vi "CameraSetupKineticSeries.vi"(1 "kinetic series pars":T1, 2 "subimage cluster":T2, 3 "error in (no error)":errorcluster, 4 "EM adv":bool) -> (5 "actual EM gain":i32, 6 "image size":cluster{"xpixels":i32, "ypixels":i32}, 7 "error out":errorcluster)   [LabVIEW 2019]
uses:
  <userlib>/atmcd32d.llb/TriggerMode_mode typedef.ctl
  <userlib>/atmcd32d.llb/AcquisitionMode_mode typedef.ctl
  <userlib>/atmcd32d.llb/ReadMode_mode typedef.ctl
  <userlib>/atmcd32d.llb/HSSpeed_type typedef.ctl
  <userlib>/atmcd32d.llb/EMGainMode_mode typedef.ctl
  GlobalCamSettingsExperiment.vi
  Global.lvlib
panel:
  out "DLL error code":u32
  out "kinetic":sgl format="%.5f"
  out "accumulate":sgl format="%.2f"
  out "exposure":sgl format="%.5f"
  out "EM gain max":i32
  out "EM gain min":i32
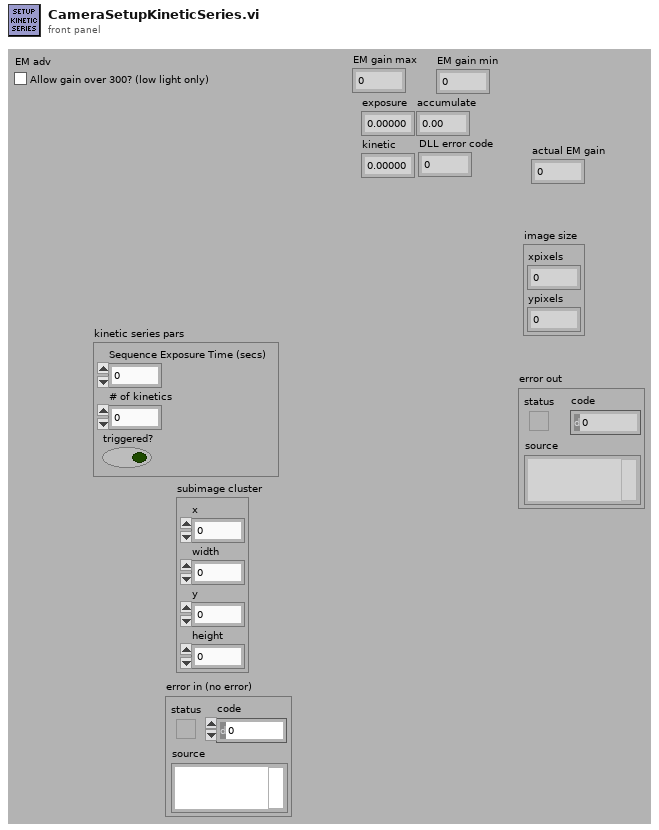
[diagram p1: front panel]
types:
  T1 = cluster{"Sequence Exposure Time (secs)":sgl, "# of kinetics":i32, "triggered?":bool}
  T2 = cluster{"x":i32, "width":i32, "y":i32, "height":i32}
  T3 = typedef "TriggerMode_mode typedef.ctl" = enum16{"Internal", "External", "N/A (2)", "N/A (3)", "N/A (4)", "N/A (5)", "External Start", "External Exposure (Bulb)", "N/A (8)", "External FVB EM", "Software", "N/A (11)", "External Charge Shifting"}
  T4 = typedef "ReadMode_mode typedef.ctl" = enum16{"Full Vertical Binning", "Multi-Track", "Random-Track", "Single-Track", "Image"}
  T5 = typedef "AcquisitionMode_mode typedef.ctl" = enum16{"Reserved (0)", "Single Scan", "Accumulate", "Kinetics", "Fast Kinetics", "Run Till Abort", "Reserved (6)", "Reserved (7)", "Reserved (8)", "Time Delayed Integration"}
  T6 = typedef "CameraSettings.ctl" = cluster{"EM Gain :":dbl, "Pre Amp Gain :":dbl, "VS Speed [Index] :":dbl, "VS Amplitude :":dbl, "Exposure Time [s] :":dbl, "Temperature :":dbl, "HS Speed [s]":dbl, "Gain > 300 :":bool}
  T7 = typedef "HSSpeed_type typedef.ctl" = enum16{"EM Amp", "Conventional Amp"}
  T8 = typedef "EMGainMode_mode typedef.ctl" = enum16{"8-bit", "12-bit", "Linear", "Real"}
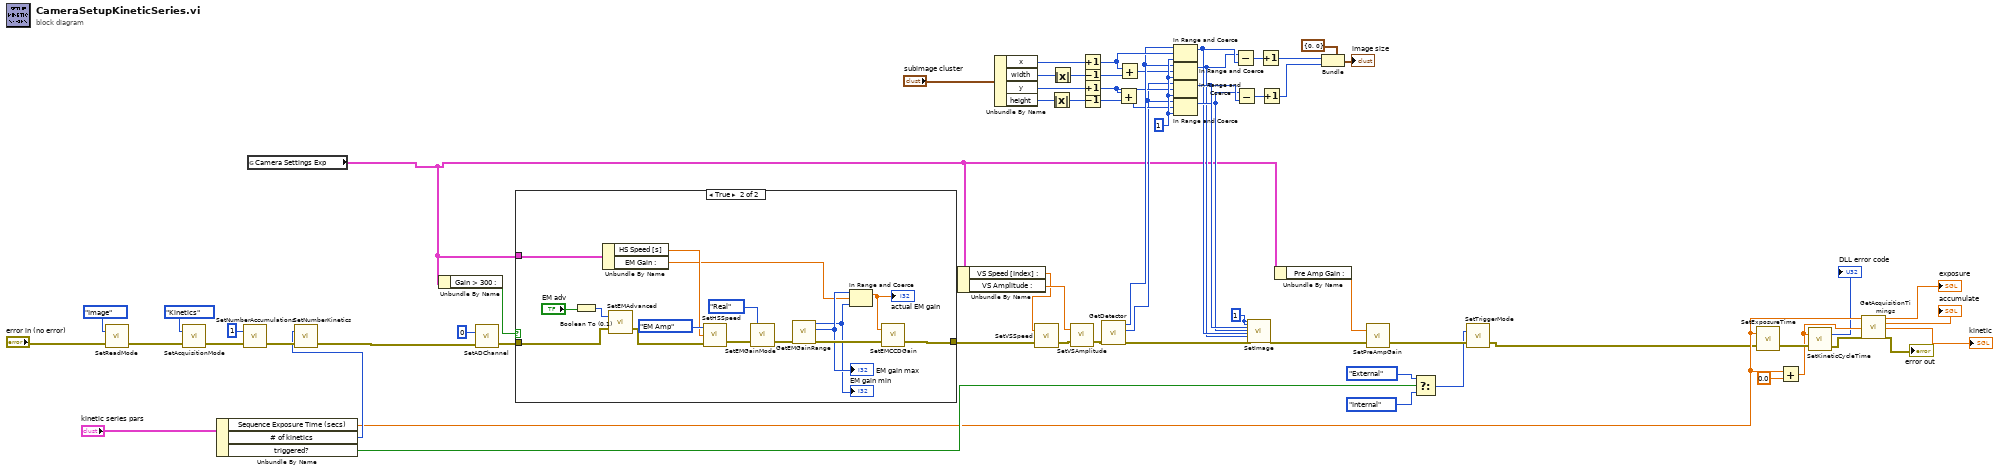
[diagram p0: block diagram]
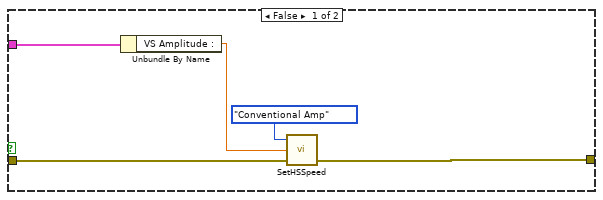
[diagram p2: hidden frame]
diagram:
  w38 = 1 ("lower limit")
  w62 = 1
  n1 = call <userlib>:"SetReadMode.vi"("error in (no error)"="error in (no error)", "mode"=ReadMode_mode_typedef."Image") -> ("error out"=w57:errorcluster)  [unwired: 1 out]
  n2 = call <userlib>:"SetAcquisitionMode.vi"("error in (no error)"=w57, "mode"=AcquisitionMode_mode_typedef."Kinetics") -> ("error out"=w50:errorcluster)  [unwired: 1 out]
  n3 = Unbundle By Name("kinetic series pars") -> ("Sequence Exposure Time (secs)"=w10:sgl, "# of kinetics"=w23:i32, "triggered?"=w16:bool)
  n4 = call <userlib>:"SetNumberAccumulations.vi"("error in (no error)"=w50, "number"=1) -> ("error out"=w48:errorcluster)  [unwired: 1 out]
  n5 = global read "GlobalCamSettingsExperiment.vi" "Camera Settings Exp"() -> (w3:T6)
  n6 = call <userlib>:"SetNumberKinetics.vi"("error in (no error)"=w48, "number"=w23) -> ("error out"=w1:errorcluster)  [unwired: 1 out]
  n7 = Unbundle By Name(w3) -> ("Gain > 300 :"=w54:bool)
  n8 = call <userlib>:"SetADChannel.vi"("error in (no error)"=w1, "channel"=0) -> ("error out"=w59:errorcluster)  [unwired: 1 out]
  n9 = case shown="True" w54 {
    tunnel: w59 -> [w69 w74]
    tunnel: [w68 w78] -> w60
    tunnel: w3 -> [w67 w77]
    frame False {
      n10 = Unbundle By Name(w67) -> ("VS Amplitude :"=w66:dbl)
      n11 = call <userlib>:"SetHSSpeed.vi"("error in (no error)"=w69, "index"=w66, "type"=HSSpeed_type_typedef."Conventional Amp") -> ("error out"=w68:errorcluster)  [unwired: 1 in, 1 out]
    }
    frame True {
      n12 = Boolean To (0,1)(Boolean="EM adv") -> (0, 1=w71:i16)
      n13 = Unbundle By Name(w77) -> ("HS Speed [s]"=w76:dbl, "EM Gain :"=w75:dbl)
      n14 = call <userlib>:"SetEMAdvanced.vi"("error in (no error)"=w74, "state"=w71) -> ("error out"=w73:errorcluster)  [unwired: 1 out]
      n15 = call <userlib>:"SetHSSpeed.vi"("error in (no error)"=w73, "index"=w76, "type"=HSSpeed_type_typedef."EM Amp") -> ("error out"=w86:errorcluster)  [unwired: 1 in, 1 out]
      n16 = call <userlib>:"SetEMGainMode.vi"("error in (no error)"=w86, "mode"=EMGainMode_mode_typedef."Real") -> ("error out"=w83:errorcluster)  [unwired: 1 out]
      n17 = call <userlib>:"GetEMGainRange.vi"("error in (no error)"=w83) -> ("error out"=w82:errorcluster, "high"=w81:i32, "low"=w80:i32)  [unwired: 3 in, 1 out]
      "EM gain max" <- w81
      "EM gain min" <- w80
      n18 = In Range and Coerce(upper limit=w81, x=w75, lower limit=w80) -> (coerced(x)=w79:dbl)  [unwired: 1 out]
      "actual EM gain" <- w79
      n19 = call <userlib>:"SetEMCCDGain.vi"("error in (no error)"=w82, "gain"=w79) -> ("error out"=w78:errorcluster)  [unwired: 1 out]
    }
  }
  n20 = Unbundle By Name(w3) -> ("VS Speed [Index] :"=w2:dbl, "VS Amplitude :"=w13:dbl)
  n21 = Unbundle By Name("subimage cluster") -> ("x"=w46:i32, "width"=w44:i32, "y"=w45:i32, "height"=w43:i32)
  n22 = call <userlib>:"SetVSSpeed.vi"("error in (no error)"=w60, "index"=w2) -> ("error out"=w15:errorcluster)  [unwired: 1 out]
  n23 = Absolute Value(x=w43) -> (abs(x)=w40:i32)
  n24 = Absolute Value(x=w44) -> (abs(x)=w33:i32)
  n25 = call <userlib>:"SetVSAmplitude.vi"("error in (no error)"=w15, "amplitude"=w13) -> ("error out"=w14:errorcluster)  [unwired: 1 out]
  n26 = Increment(x=w46) -> (x+1=w39:i32)
  n27 = Decrement(x=w33) -> (x-1=w42:i32)
  n28 = Increment(x=w45) -> (x+1=w35:i32)
  n29 = Decrement(x=w40) -> (x-1=w41:i32)
  n30 = call <userlib>:"GetDetector.vi"("error in (no error)"=w14) -> ("error out"=w61:errorcluster, "ypixels"=w32:i32, "xpixels"=w37:i32)  [unwired: 3 in, 1 out]
  n31 = Add(x=w35, y=w41) -> (x+y=w34:i32)
  n32 = Add(x=w39, y=w42) -> (x+y=w36:i32)
  n33 = In Range and Coerce(upper limit=w37, x=w39, lower limit=w38) -> (coerced(x)=w25:i32)  [unwired: 1 out]
  n34 = In Range and Coerce(upper limit=w37, x=w36, lower limit=w38) -> (coerced(x)=w24:i32)  [unwired: 1 out]
  n35 = In Range and Coerce(upper limit=w32, x=w35, lower limit=w38) -> (coerced(x)=w27:i32)  [unwired: 1 out]
  n36 = In Range and Coerce(upper limit=w32, x=w34, lower limit=w38) -> (coerced(x)=w26:i32)  [unwired: 1 out]
  n37 = Subtract(x=w24, y=w25) -> (x-y=w31:i32)
  n38 = Subtract(x=w26, y=w27) -> (x-y=w29:i32)
  n39 = call <userlib>:"SetImage.vi"("hbin"=w62, "vbin"=w62, "hstart"=w27, "hend"=w26, "vstart"=w25, "vend"=w24, "error in (no error)"=w61) -> ("error out"=w63:errorcluster)  [unwired: 19 in, 1 out]
  n40 = Increment(x=w31) -> (x+1=w30:i32)
  n41 = Increment(x=w29) -> (x+1=w28:i32)
  n42 = Unbundle By Name(w3) -> ("Pre Amp Gain :"=w53:dbl)
  n43 = Bundle(cluster=cluster{"xpixels":i32, "ypixels":i32} {"xpixels"=0, "ypixels"=0} ("image size"), "xpixels"=w30, "ypixels"=w28) -> (→"image size":cluster{"xpixels":i32, "ypixels":i32})
  n44 = call <userlib>:"SetPreAmpGain.vi"("error in (no error)"=w63, "index"=w53) -> ("error out"=w64:errorcluster)  [unwired: 1 out]
  n45 = Select(t=TriggerMode_mode_typedef."External" ("mode"), s=w16, f=TriggerMode_mode_typedef."Internal" ("mode")) -> (s? t:f=w17:T3)
  n46 = call <userlib>:"SetTriggerMode.vi"("error in (no error)"=w64, "mode"=w17) -> ("error out"=w5:errorcluster)  [unwired: 1 out]
  n47 = call <userlib>:"SetExposureTime.vi"("error in (no error)"=w5, "time"=w10) -> ("error out"=w22:errorcluster)  [unwired: 1 out]
  n48 = Add(x=w10, y=sgl 0.0) -> (x+y=w9:sgl)
  n49 = call <userlib>:"SetKineticCycleTime.vi"("error in (no error)"=w22, "time"=w9) -> ("error out"=w12:errorcluster, "DLL error code"=→"DLL error code":u32)
  n50 = call <userlib>:"GetAcquisitionTimings.vi"("exposure input"=w10, "kinetic input"=w9, "error in (no error)"=w12) -> ("exposure"=→"exposure":sgl, "accumulate"=→"accumulate":sgl, "kinetic"=→"kinetic":sgl, "error out"=→"error out":errorcluster)  [unwired: 8 in, 1 out]
